vi "Win32 Parse MIB_FORWARDROW.vi"(11 "pBestRoute":u32[](array[numeric])) -> (1 "prefix":i32, 2 "address out":refnum<class "Generic Network Address.lvclass">, 3 "network":refnum<class "Generic Network Address.lvclass">)   [LabVIEW 2020, in "NI_WFCN.lvlib" / "IPv4 Network Address.lvclass"]
doc: "Parse a Win32 MIB_FORWARDROW data structure, such as is returned by GetBestRoute to determine if an IPv4 address is routable."
uses:
  <vilib>/net/WFCN/Addressing/IPv4 Network Address/IPv4 Network Address.lvclass
  <vilib>/net/WFCN/Addressing/Generic Network Address/Generic Network Address.lvclass
  <vilib>/net/WFCN/Addressing/IPv4 Network Address/IPv4 Network Address.lvclass/IPv4 Network Address.ctl
  e:/builds/penguin/labview/branches/2020/dev/dist/vi.lib/net/WFCN/Addressing/Generic Network Address/Generic Network Address.lvclass
  <vilib>/net/WFCN/NI_WFCN.lvlib
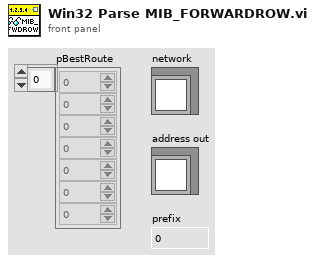
[diagram p1: front panel]
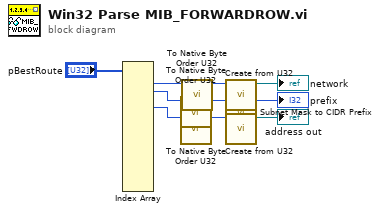
[diagram p0: block diagram]
diagram:
  n1 = Index Array(array="pBestRoute") -> (element #1=w3:u32, element #2=w1:u32, element #4=w5:u32)  [unwired: 14 in, 11 out]
  n2 = call <vilib>:"To Native Byte Order U32.vi"("network byte order"=w1) -> ("native byte order"=w2:u32)  [unwired: 6 in]
  n3 = call <vilib>:"To Native Byte Order U32.vi"("network byte order"=w5) -> ("native byte order"=w6:u32)  [unwired: 6 in]
  n4 = call <vilib>:"To Native Byte Order U32.vi"("network byte order"=w3) -> ("native byte order"=w4:u32)  [unwired: 6 in]
  n5 = call <vilib>:"Create from U32.vi"("address U32"=w4) -> ("address out"=→"network":refnum<class "IPv4 Network Address.lvclass">)  [unwired: 10 in]
  n6 = call <vilib>:"Subnet Mask to CIDR Prefix.vi"("address"=w2) -> ("prefix"=→"prefix":i32)  [unwired: 6 in]
  n7 = call <vilib>:"Create from U32.vi"("address U32"=w6) -> ("address out"=→"address out":refnum<class "IPv4 Network Address.lvclass">)  [unwired: 10 in]
